vi "Prober_InitObject.vi"(8 "error in (no error)":errorcluster, 10 "Prober Configuration":variant, 11 "SemiProbe in":refnum<class "SemiProbe.lvclass">) -> (0 "error out":errorcluster, 3 "SemiProbe out":refnum<class "SemiProbe.lvclass">)   [LabVIEW 2018, in "SemiProbe.lvclass"]
uses:
  SemiProbe.lvclass
  SemiProbe.vi
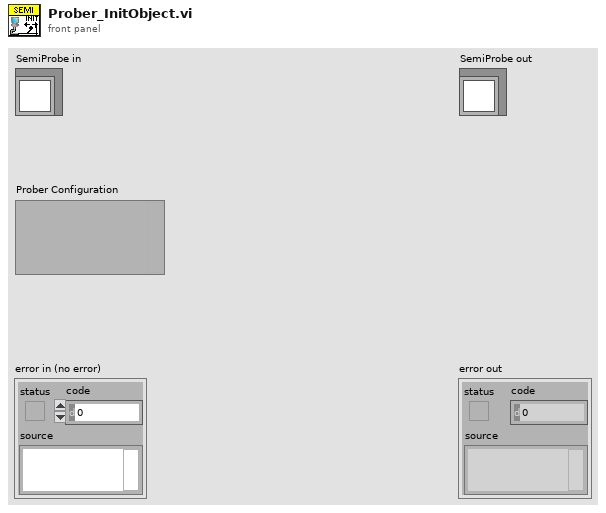
[diagram p1: front panel]
types:
  T1 = cluster{"SP Local":bool, "SP Min Usable Z":dbl, "SP REMOTE Comm Parameters":cluster{"SemiProbe VISA":refnum<visa-resource-name>, "write delay(ms)":i32, "buffer is full loop multiplicity":i32, "read threshold check rate (ms)":u32}, "SP Comm Params":cluster{"LF as Return EOL":bool, "SP Error Debug":bool}, "SP LOCAL Comm Parameters":cluster{"address":string, "port":i32, "SP TCP Cnx ID":refnum<k5>, "mode (standard)":enum16{"Standard", "Buffered", "CRLF", "Immediate"}, "bytes to read":i32, "timeout (ms)":i32}, "SP Operation Parameters":cluster{"SP Load Less Than Thr?":bool, "SP Load Threshold (um)":dbl, "SP Current Location":cluster{"X (um)":ext, "Y (um)":ext, "Z (um)":ext, "T (degree)":ext}, "SP Chuck Speeds":cluster{"XY Speed (10-100%)":dbl, "Z Speed (10-100%)":dbl, "T Speed (10-100%)":dbl}, "Manual Step Parameters":cluster{"Step in X":bool, "X S-Speed [µm/step]":sgl, "Step in Y":bool, "Y S-Speed [µm/step]":sgl, "Step in Z":bool, "Z S-Speed [µm/step]":sgl, "Step in T":bool, "T S-Speed [mdegree/step]":sgl, "X Increase":bool, "Y Increase?":bool, "Z Increase?":bool, "T Increase?":bool}, "Z Stepper":cluster{"UP/DOWN":bool, "UP/DOWN Speed [µm/step]":i32, "SP Z Step":bool}, "Z Heights Set":bool, "SP Contact Search":cluster{"Contact Circuit":enum16{"12", "1", "2"}, "Speed [1000-10000]":sgl, "Start Height [µm]":sgl, "Search Band [µm]":sgl, "Overdrive [µm]":sgl}, "Separation Distance [µm]":u32, "Contact Height [µm]":u32, "Use Overdrive?":bool, "Touchdown method":enum16{"no feedback", "Arduino edgesense", "SP contact circuit"}, "Arduino Edgesense params":cluster{"touchdown height [µm]":i32, "search band [µm]":u32, "speed [µm/step]":u32, "overdrive [µm]":u32}}}
  T2 = cluster{"SemiProbe VISA":refnum<visa-resource-name>, "write delay(ms)":i32, "buffer is full loop multiplicity":i32, "read threshold check rate (ms)":u32}
  T3 = cluster{"address":string, "port":i32, "SP TCP Cnx ID":refnum<k5>, "mode (standard)":enum16{"Standard", "Buffered", "CRLF", "Immediate"}, "bytes to read":i32, "timeout (ms)":i32}
  T4 = cluster{"SP Load Less Than Thr?":bool, "SP Load Threshold (um)":dbl, "SP Current Location":cluster{"X (um)":ext, "Y (um)":ext, "Z (um)":ext, "T (degree)":ext}, "SP Chuck Speeds":cluster{"XY Speed (10-100%)":dbl, "Z Speed (10-100%)":dbl, "T Speed (10-100%)":dbl}, "Manual Step Parameters":cluster{"Step in X":bool, "X S-Speed [µm/step]":sgl, "Step in Y":bool, "Y S-Speed [µm/step]":sgl, "Step in Z":bool, "Z S-Speed [µm/step]":sgl, "Step in T":bool, "T S-Speed [mdegree/step]":sgl, "X Increase":bool, "Y Increase?":bool, "Z Increase?":bool, "T Increase?":bool}, "Z Stepper":cluster{"UP/DOWN":bool, "UP/DOWN Speed [µm/step]":i32, "SP Z Step":bool}, "Z Heights Set":bool, "SP Contact Search":cluster{"Contact Circuit":enum16{"12", "1", "2"}, "Speed [1000-10000]":sgl, "Start Height [µm]":sgl, "Search Band [µm]":sgl, "Overdrive [µm]":sgl}, "Separation Distance [µm]":u32, "Contact Height [µm]":u32, "Use Overdrive?":bool, "Touchdown method":enum16{"no feedback", "Arduino edgesense", "SP contact circuit"}, "Arduino Edgesense params":cluster{"touchdown height [µm]":i32, "search band [µm]":u32, "speed [µm/step]":u32, "overdrive [µm]":u32}}
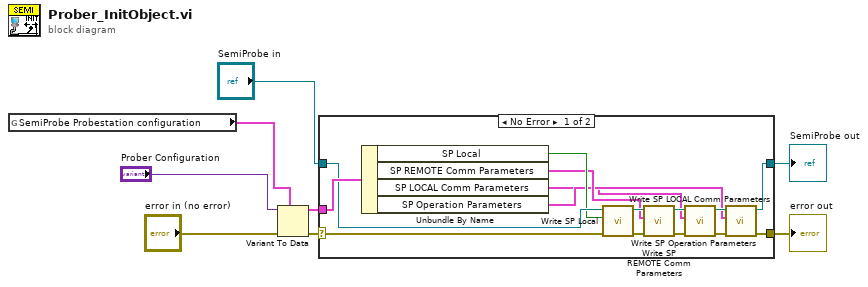
[diagram p0: block diagram]
diagram:
  n1 = global read "SemiProbe.vi" "SemiProbe Probestation configuration"() -> (w1:T1)
  n2 = Variant To Data(error in="error in (no error)", type=w1, Variant="Prober Configuration") -> (data=w3:T1, error out=w5:errorcluster)
  n3 = case shown="No Error" w5 {
    selector: w5 -> [w21 w25]
    tunnel: "SemiProbe in" -> [w22 w24]
    tunnel: [w12 w25] -> w8
    tunnel: [w11 w24] -> w7
    tunnel: w3 -> [w23 _]
    frame No Error {
      n4 = Unbundle By Name(w23) -> ("SP Local"=w20:bool, "SP REMOTE Comm Parameters"=w18:T2, "SP LOCAL Comm Parameters"=w9:T3, "SP Operation Parameters"=w10:T4)
      n5 = call-dynamic "Write SP Local.vi"("error in (no error)"=w21, "SP Local"=w20, "SemiProbe in"=w22) -> ("error out"=w17:errorcluster, "SemiProbe out"=w19:refnum<class "SemiProbe.lvclass">)  [unwired: 7 in]
      n6 = call-dynamic "Write SP REMOTE Comm Parameters.vi"("error in (no error)"=w17, "SP REMOTE Comm Parameters"=w18, "SemiProbe in"=w19) -> ("error out"=w15:errorcluster, "SemiProbe out"=w16:refnum<class "SemiProbe.lvclass">)  [unwired: 7 in]
      n7 = call-dynamic "Write SP LOCAL Comm Parameters.vi"("error in (no error)"=w15, "SP LOCAL Comm Parameters"=w9, "SemiProbe in"=w16) -> ("error out"=w13:errorcluster, "SemiProbe out"=w14:refnum<class "SemiProbe.lvclass">)  [unwired: 7 in]
      n8 = call-dynamic "Write SP Operation Parameters.vi"("error in (no error)"=w13, "SP Operation Parameters"=w10, "SemiProbe in"=w14) -> ("error out"=w12:errorcluster, "SemiProbe out"=w11:refnum<class "SemiProbe.lvclass">)  [unwired: 7 in]
    }
    frame Error {
    }
  }
  "error out" <- w8
  "SemiProbe out" <- w7
